vi "cRIO_4DoF_Gonio_forward_kinematics.vi"(0 "X in":cdb, 5 "Y in":cdb, 7 "Z in":cdb, 11 "Theta6_meas":dbl) -> (4 "X out":dbl, 6 "Y out":dbl, 8 "Z out":dbl, 10 "yaw":dbl, 15 "RGonimeter":dbl[][](array[numeric]))   [LabVIEW 2019]
uses:
  Global 1.vi
  <vilib>/imath/engines/lvmath2/RunTimeEngine/Managers/WorkSpace/UID Generator.vi
  <vilib>/imath/engines/lvmath2/RunTimeEngine/ArithmeticOperatorToken/NIMS_ArithmeticOperator_multmx-internal.vi
  <instcachedir>/0/NIMS_ArithmeticOperator_multmx-internal_9E91BA3A2DCB4083AAD724A04442A6F7.lvgen/NIMS_ArithmeticOperator_multmx-internal_9E91BA3A2DCB4083AAD724A04442A6F7_004.vi
  <vilib>/imath/engines/lvmath2/RunTimeEngine/ErrorHandling/NIMS_Create Error From Enums.vi
  <vilib>/imath/engines/lvmath2/RunTimeEngine/IndexRead/NIMS M(S,S).vi
  <instcachedir>/0/NIMS M(S,S)_AC51E74150A542F7991B9634C66F3096.lvgen/NIMS M(S,S)_AC51E74150A542F7991B9634C66F3096_000.vi
  <vilib>/imathl/engines/lvmath/Functions/Error Handling/Create Error.vi
  <vilib>/imath/engines/lvmath2/RunTimeEngine/IndexRead/NIMS M(R2,R2).vi
  <instcachedir>/0/NIMS M(R2,R2)_A604CBC2A3B94D18B31C03B21D5CD7AA.lvgen/NIMS M(R2,R2)_A604CBC2A3B94D18B31C03B21D5CD7AA_000.vi
  <vilib>/imath/engines/lvmath2/RunTimeEngine/RunTimeType/NIMS_RunTimeType_From StrictType (excl LVString).vi
  <instcachedir>/0/NIMS_RunTimeType_From StrictType (excl LVString)_D8AFBA86A94845AAA577C895450664BD.lvgen/NIMS_RunTimeType_From StrictType (excl LVString)_D8AFBA86A94845AAA577C895450664BD_000.vi
  <vilib>/imath/engines/lvmath2/RunTimeEngine/LocalVariableDefStatement/MC_LocalVariableDefStatement_Display.vi
  <vilib>/imath/engines/lvmath2/RunTimeEngine/Managers/SymbolTable/Clear UID.vi
  <vilib>/imath/engines/lvmath2/RunTimeEngine/NodeEndStatement/NIMS_NodeEndStatement_Output.vi
  <instcachedir>/0/NIMS_NodeEndStatement_Output_53EC0D466D134D7ABD903AC30B43404B.lvgen/NIMS_NodeEndStatement_Output_53EC0D466D134D7ABD903AC30B43404B_001.vi
  <instcachedir>/0/NIMS_NodeEndStatement_Output_53EC0D466D134D7ABD903AC30B43404B.lvgen/NIMS_NodeEndStatement_Output_53EC0D466D134D7ABD903AC30B43404B_002.vi
  <vilib>/imath/engines/lvmath2/RunTimeEngine/ErrorHandling/NIMS_Finalize Error.vi
  <vilib>/imath/engines/lvmath2/RunTimeEngine/Managers/SymbolTable/NIMS_WorkSpace.lvlib
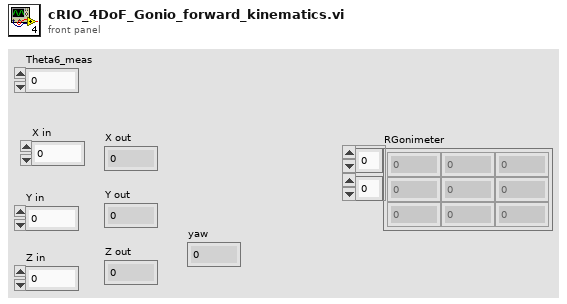
[diagram p1: front panel]
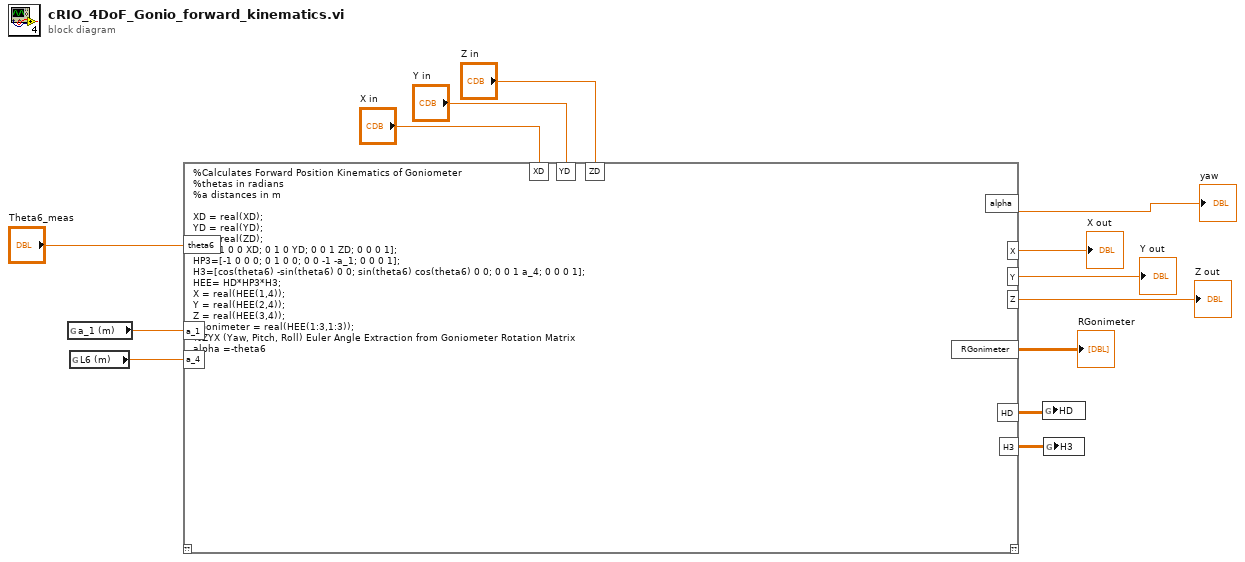
[diagram p0: block diagram]
diagram:
  n1 = global read "Global 1.vi" "a_1 (m)"() -> (w4:dbl)
  n2 = global read "Global 1.vi" "L6 (m)"() -> (w3:dbl)
  n3 = mathscript code="%Calculates Forward Position Kinematics of Goniometer\n%thetas in radians\n%a distances in m\n\nXD = real(XD);\nYD = real(YD);\nZD = real(ZD);\nHD=[1 0 0 XD; 0 1 0 YD; 0 0 1 ZD; 0 0 0 1];\nHP3=[-1 0 0 0; 0 1 0 0; 0 0 -1 -a_1; 0 0 0 1];\nH3=[cos(theta6) -sin(theta6) 0 0; sin(theta6) cos(theta6) 0 0; 0 0 1 a_4; 0 0 0 1];\nHEE= HD*HP3*H3; \nX = real(HEE(1,4));\nY = real(HEE(2,4));\nZ = real(HEE(3,4));\nRGonimeter = real(HEE(1:3,1:3));\n%ZYX (Yaw, Pitch, Roll) Euler Angle Extraction from Goniometer Rotation Matrix\nalpha =-theta6"("a_1"=w4, "a_4"=w3, "theta6"="Theta6_meas", "XD"="X in", "YD"="Y in", "ZD"="Z in") -> ("X"=→"X out":dbl, "Y"=→"Y out":dbl, "Z"=→"Z out":dbl, "RGonimeter"=→"RGonimeter":dbl[][], "HD"=w2:dbl[][], "H3"=w1:dbl[][], "alpha"=→"yaw":dbl)  [unwired: 1 in, 1 out]
  n4 = global write "Global 1.vi" "HD"(w2) -> ()
  n5 = global write "Global 1.vi" "H3"(w1) -> ()
